vi "Update room Size.vi"(0 "Guest Manager Model in":refnum<class "Guest Manager Model.lvclass">, 5 "Room Sizes":string[](array[string]), 11 "error in (no error)":errorcluster) -> (4 "Guest Manager Model out":refnum<class "Guest Manager Model.lvclass">, 15 "error out":errorcluster)   [LabVIEW 2023, in "Guest Manager Model.lvlib" / "Guest Manager Model.lvclass"]
uses:
  Guest Manager Model.lvclass
  <vilib>/ActorFramework/Actor/Actor.lvclass/Actor.ctl
  <vilib>/ActorFramework/Message Enqueuer/Message Enqueuer.lvclass/Message Enqueuer.ctl
  Guest Manager UI/Guest Manager UI Messages/Update Room Size Msg/Update Room Size Msg.lvclass/Update Room Size Msg.ctl
  <vilib>/ActorFramework/Message Enqueuer/Init from Existing Queue.vi
  <vilib>/ActorFramework/Message Enqueuer/Enqueue.vi
  Guest Manager UI/Guest Manager UI Messages/Update Room Size Msg/Update Room Size Msg.lvclass
  <vilib>/ActorFramework/Message Priority Queue/Priority Enqueue.vi
  <vilib>/ActorFramework/Message Enqueuer/Message Enqueuer.lvclass
  Guest Manager Model.lvclass/Guest Manager Model.ctl
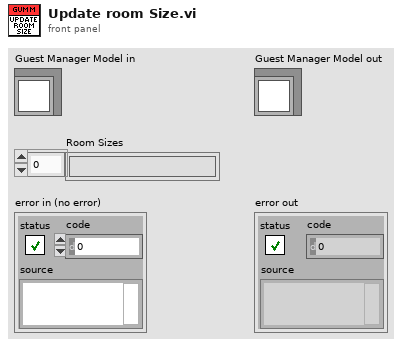
[diagram p1: front panel]
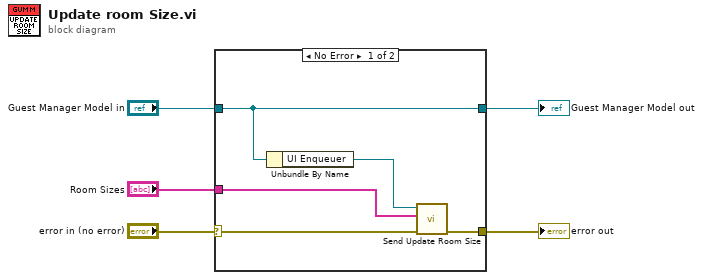
[diagram p0: block diagram]
diagram:
  n1 = case shown="No Error" "error in (no error)" {
    selector: "error in (no error)" -> [w10 w12]
    tunnel: [w9 w12] -> w4
    tunnel: [w7 w11] -> w2
    tunnel: "Guest Manager Model in" -> [w7 w11]
    tunnel: "Room Sizes" -> [w8 _]
    frame No Error {
      n2 = Unbundle By Name(w7) -> ("UI Enqueuer"=w6:refnum<class "Message Enqueuer.lvclass">)
      n3 = call "Send Update Room Size.vi"("error in (no error)"=w10, "Room Sizes"=w8, "Message Enqueuer"=w6) -> ("error out"=w9:errorcluster)  [unwired: 7 in, 1 out]
    }
    frame Error {
    }
  }
  "error out" <- w4
  "Guest Manager Model out" <- w2
